vi "calc_similarity.vi"(1 "data2":dbl[][](array[numeric])=[[0.0, 1.0, 0.4, 2.0, 5.0, 1.0, 0.0, 0.0], [5.0, 2.0, 0.45, 2.1, 5.5, 1.0, 0.0, 0.0], [6.0, 0.8, 0.35, 2.0, 1.0, 5.0, 0.0, -1.0]], 2 "Detector in":refnum<class "Detector.lvclass">, 3 "data1":dbl[][](array[numeric])=[[0.0, 1.0, 0.4, 2.0, 5.0, 1.0, 0.0, 0.0], [5.0, 2.0, 0.45, 2.1, 5.5, 1.0, 0.0, 0.0], [6.0, 0.8, 0.35, 2.0, 1.0, 5.0, 0.0, -1.0]]) -> (0 "res out":i32[](array[numeric]))   [LabVIEW 2020, in "Detector.lvclass"]
uses:
  Detector.lvclass
  Detector.lvclass/Detector.ctl
  dependecies/globalVarII.vi
  dependecies/globalVarSD.vi
panel:
  out "error out":errorcluster
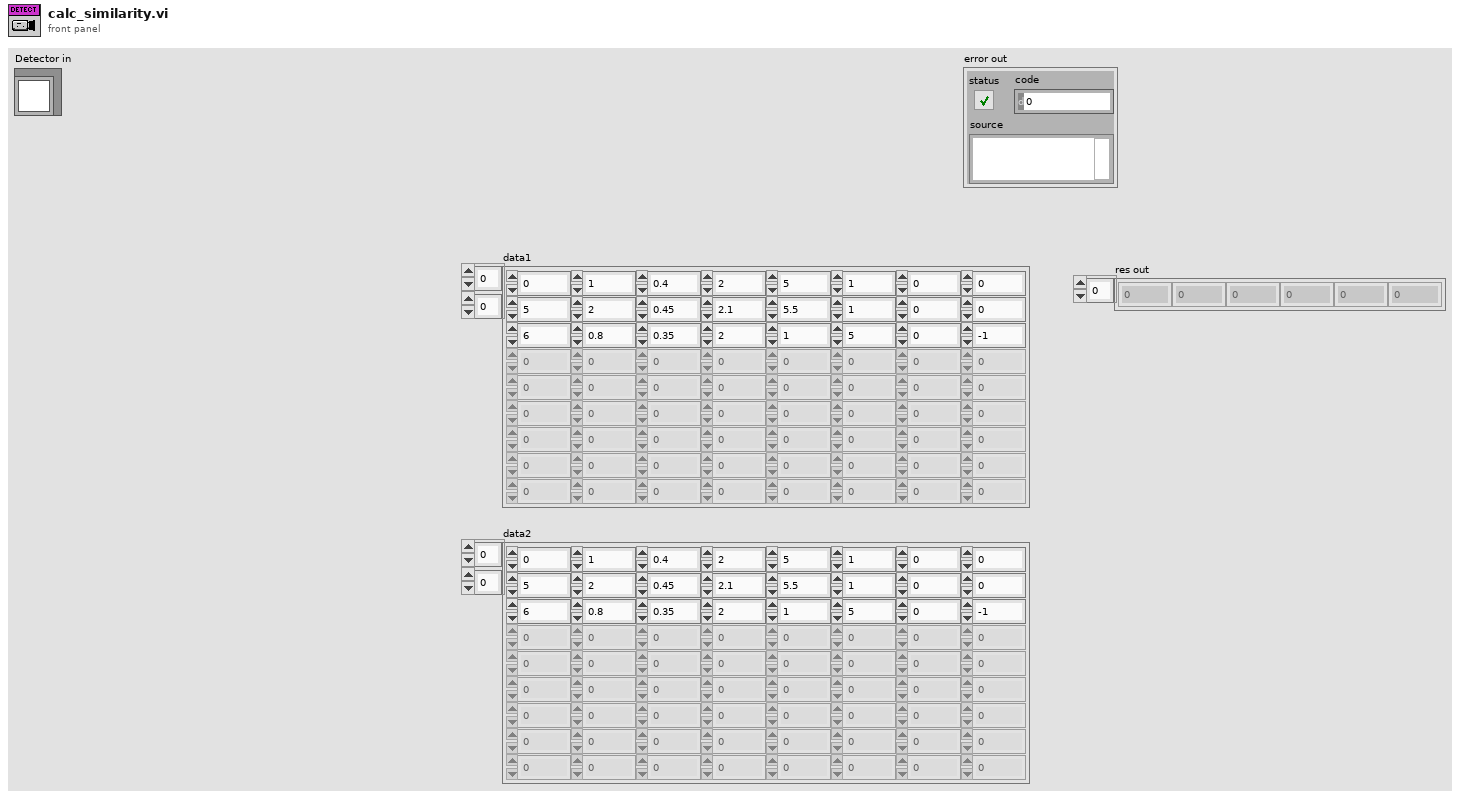
[diagram p1: front panel]
types:
  T1 = typedef "Control-Client.lvclass/Controls-refs_CLIENT.ctl" = cluster{"ON/OFF Cool":refnum<vi>, "Save spectra":refnum<vi>, "Read detector":refnum<vi>, "# scans":refnum<vi>, "BG-level":refnum<vi>, "Set T":refnum<vi>, "Termometer":refnum<vi>, "Spectra":refnum<vi>, "Error Meter_ref":refnum<vi>, "OD graph":refnum<vi>, "from_pixel":refnum<vi>, "to_pixel":refnum<vi>, "threshold_ref_channel":refnum<vi>, "value":refnum<vi>, "python session":refnum<vi>, "ref h5_file":T2, "distance":refnum<vi>}
  T2 = typedef "hid_t.ctl" = i64
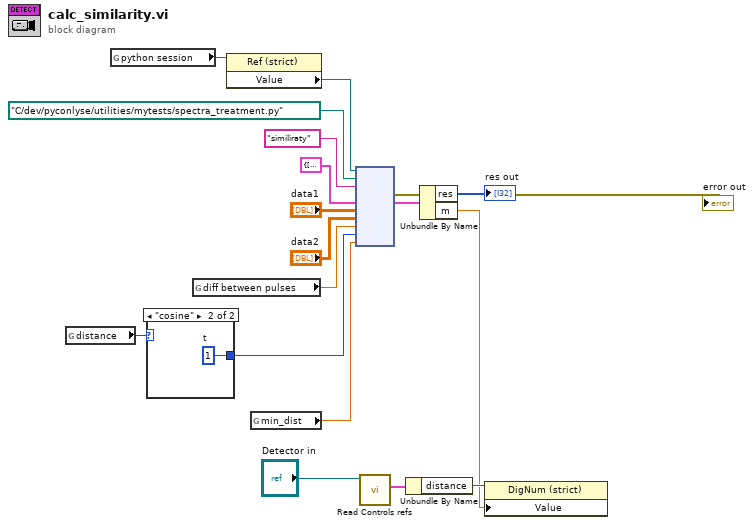
[diagram p0: block diagram]
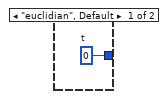
[diagram p2: hidden frame]
diagram:
  n1 = global read "globalVarII.vi" "distance"() -> (w8:enum32{"euclidian", "cosine"})
  n2 = global read "globalVarSD.vi" "python session"() -> (w9:refnum<vi>)
  n3 = case shown="\"cosine\"" w8 {
    tunnel: [w19 w20] -> w7
    frame "euclidian", Default {
      w19 = 0  # t
    }
    frame "cosine" {
      w20 = 1  # t
    }
  }
  n4 = global read "globalVarII.vi" "diff between pulses"() -> (w14:dbl)
  n5 = property class="Ref (strict)"(reference=w9) -> ("Value"=w17:refnum<k35>)  [unwired: 1 in, 2 out]
  n6 = global read "globalVarII.vi" "min_dist"() -> (w6:dbl)
  n7 = node(w17, path "C:/dev/pyconlyse/utilities/mytests/spectra_treatment.py" ("module path"), "similiraty" ("function name"), cluster{"res":i32[], "m":dbl} {"res"=[], "m"=0.0}, "data1", "data2", w14, w7, w6) -> (→"error out":errorcluster, w11:cluster{"res":i32[], "m":dbl})  [unwired: 6 in, 3 out]
  n8 = call "Read Controls refs.vi"("Detector in"="Detector in") -> ("Controls refs"=w4:T1)  [unwired: 8 in, 2 out]
  n9 = Unbundle By Name(w4) -> ("distance"=w3:refnum<vi>)
  n10 = Unbundle By Name(w11) -> ("res"=→"res out":i32[], "m"=w2:dbl)
  n11 = property class="DigNum (strict)"(reference=w3, "Value"=w2) -> ()  [unwired: 1 in, 2 out]
